vi "ProducerConsumerDAQ.vi"() -> ()   [LabVIEW 2014]
doc: "Use this template to build a user interface event handler design pattern. Use this pattern for dialog boxes and other user interfaces. You also can create and execute user-defined events that the VI can handle the same way as user interface events."
uses:
  subVIs/MasterState.ctl
  subVIs/SlaveStateData.ctl
  subVIs/SlaveState.ctl
  <vilib>/Utility/error.llb/DialogType.ctl
  <vilib>/DAQmx/create/channels.llb/DAQmx Create Channel (AI-Voltage-Basic).vi
  <vilib>/DAQmx/configure/timing.llb/DAQmx Timing (Sample Clock).vi
  <vilib>/DAQmx/read.llb/DAQmx Read (Analog Wfm 1Chan NSamp).vi
  <resource>/objmgr/daqmx.rc
panel:
  in  "File Path":path
  in  "Acquire Data":bool
  in  "Log Data":bool
  in  "File Comment":string
  in  "DAQ Parameters":T1={"physical channels"="", "maximum value"=5.0, "minimum value"=-5.0, "rate"=1000.0, "read period"=0.5} {"read period" format="%0.2f"; "rate" format="%0.2f"; "minimum value" format="%0.2f"; "maximum value" format="%0.2f"}
  out "Waveform Chart":waveform(dbl)(graph)
  in  "quit":bool
  # "V"
  # "V"
  # "Hz"
  # "s"
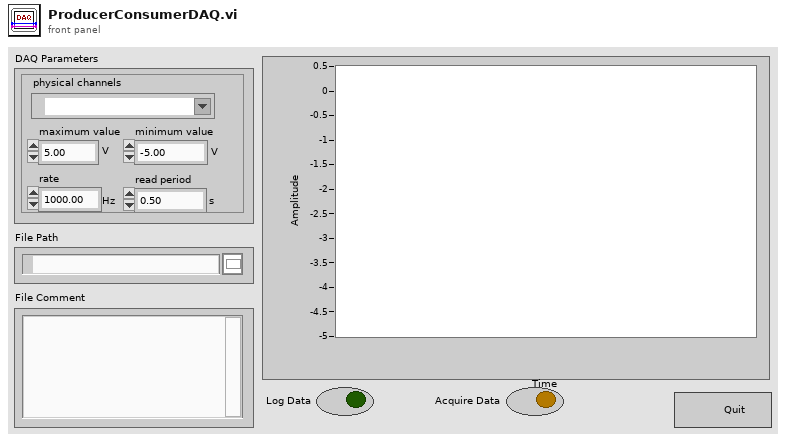
[diagram p1: front panel]
types:
  T1 = cluster{"physical channels":tag, "maximum value":dbl, "minimum value":dbl, "rate":dbl, "read period":dbl}
  T2 = typedef "SlaveState.ctl" = enum16{"Init", "Idle", "CheckError", "Finalize", "StartDAQ", "AcquireAndLog", "StopDAQ", "UpdateFile"}
  T3 = typedef "SlaveStateData.ctl" = cluster{"New State":T2, "DAQ Ref":refnum<k21>, "File Ref":refnum<file>}
  T4 = typedef "MasterState.ctl" = enum16{"Init", "Idle", "CheckError", "Finalize", "ConfigDAQ", "StartDAQ", "AcquireAndLog", "StopDAQ", "ClearDAQ", "OpenFile", "CloseFile"}
  T5 = typedef "DialogType.ctl" = u16
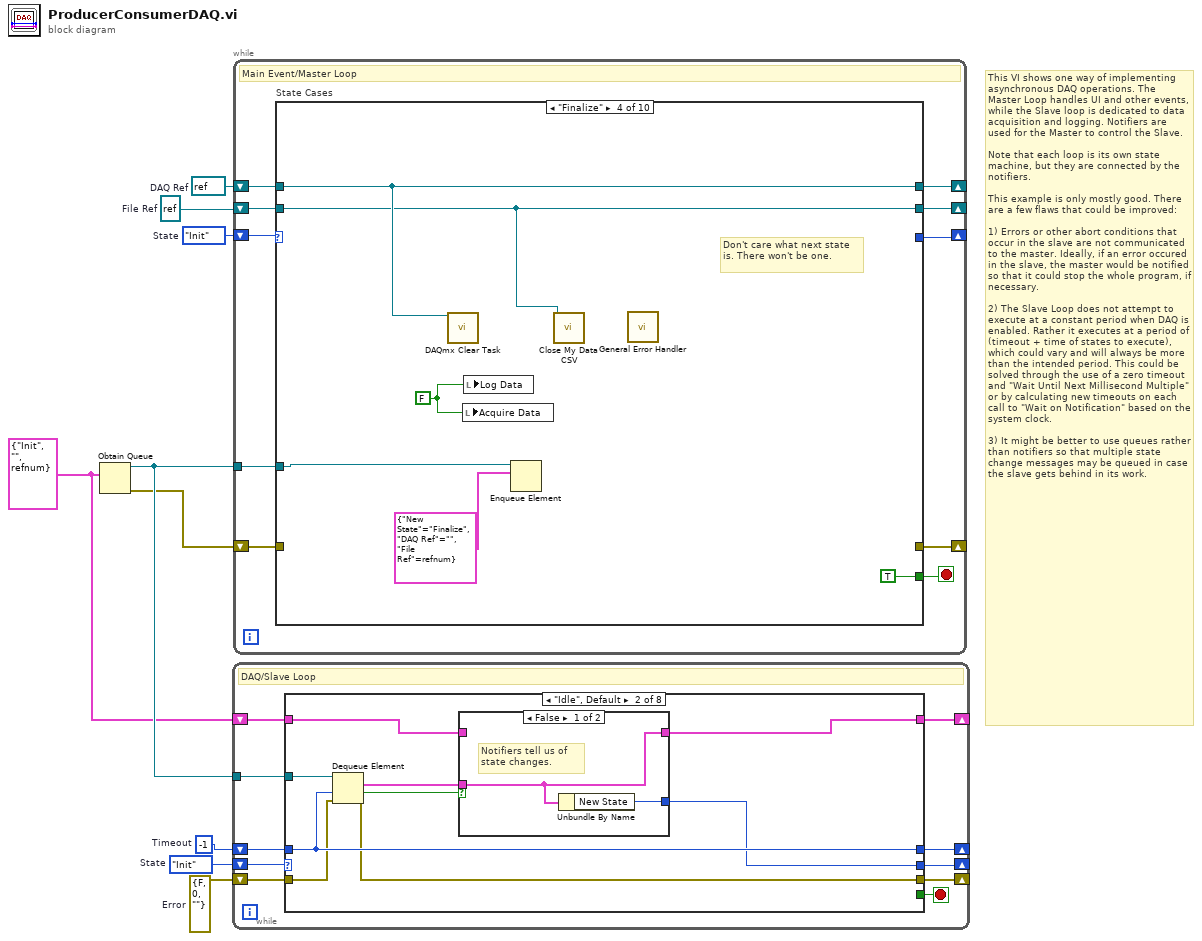
[diagram p0: block diagram]
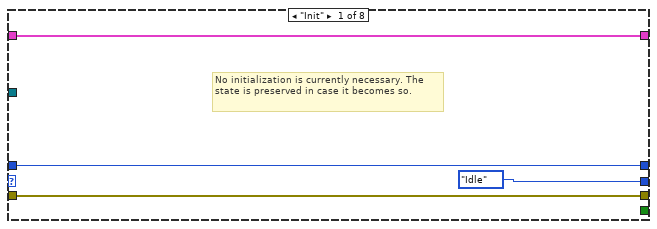
[diagram p2: hidden frame]
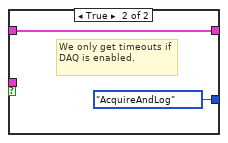
[diagram p3: hidden frame]
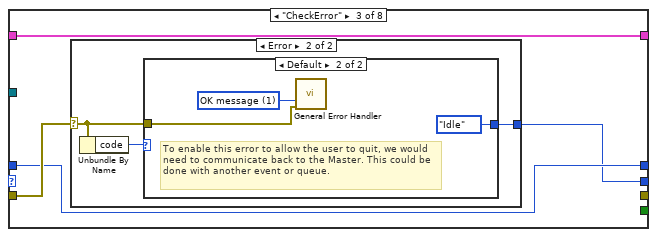
[diagram p4: hidden frame]
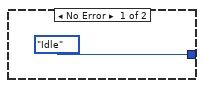
[diagram p5: hidden frame]
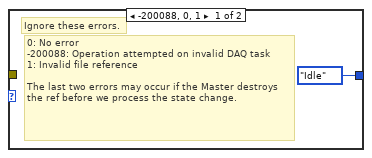
[diagram p6: hidden frame]
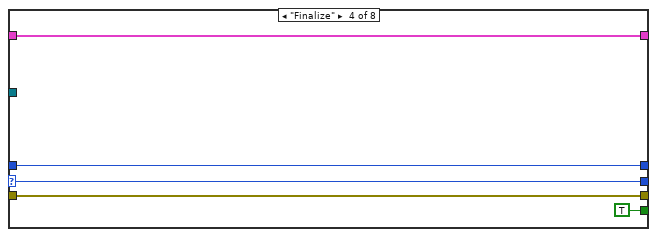
[diagram p7: hidden frame]
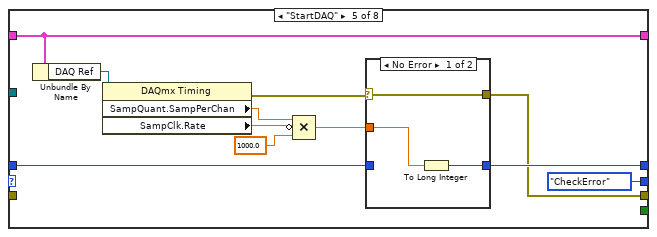
[diagram p8: hidden frame]
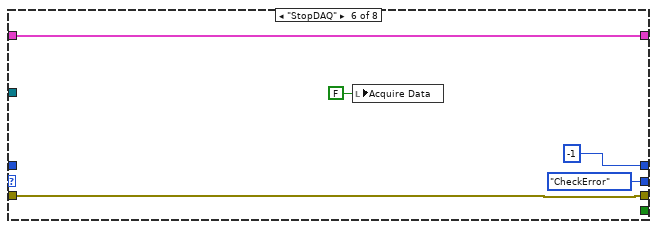
[diagram p10: hidden frame]
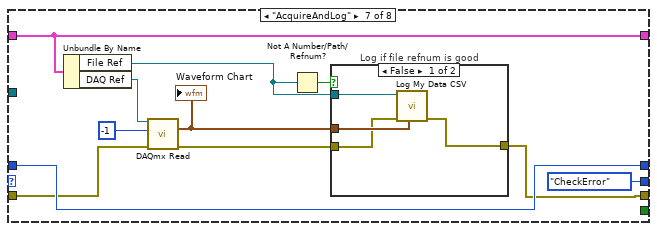
[diagram p11: hidden frame]
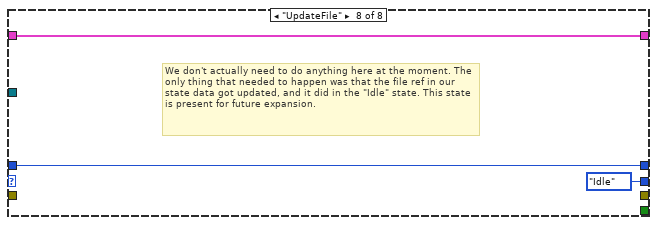
[diagram p13: hidden frame]
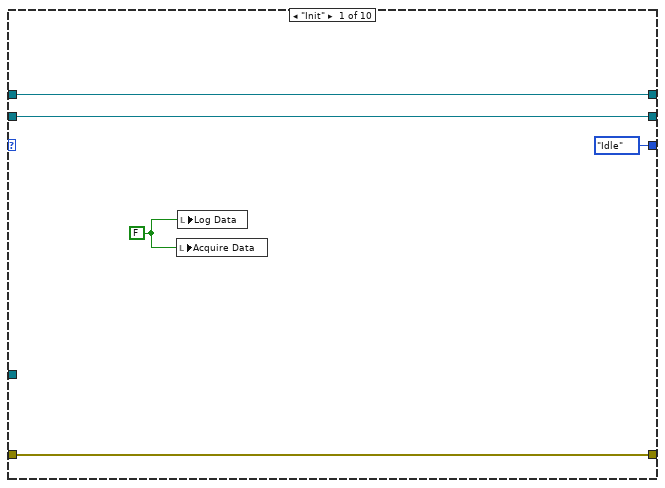
[diagram p14: hidden frame]
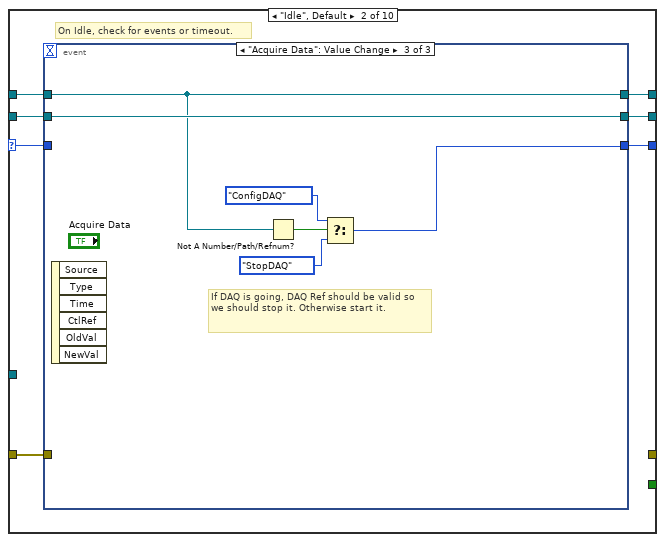
[diagram p15: hidden frame]
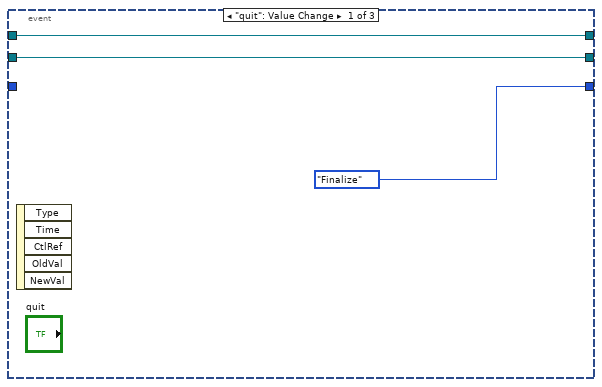
[diagram p16: hidden frame]
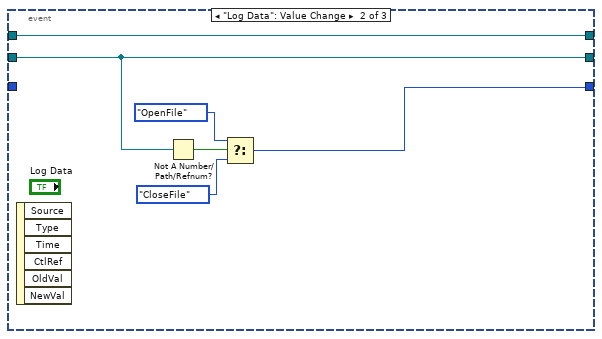
[diagram p17: hidden frame]
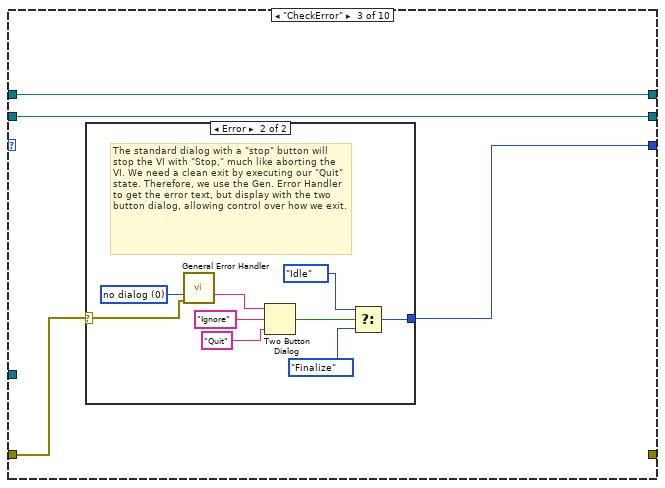
[diagram p18: hidden frame]
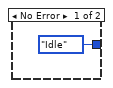
[diagram p19: hidden frame]
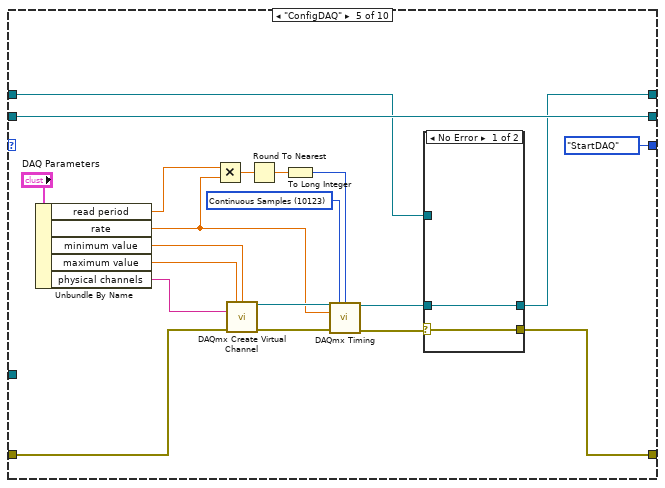
[diagram p20: hidden frame]
diagram:
  w1 = errorcluster {"status"=FALSE, "code"=0, "source"=""}  # Error
  w3 = -1  # Timeout
  w5 = SlaveState."Init"  # State
  w4 = T3 {"New State"=enum."Init", "DAQ Ref"="", "File Ref"=refnum}
  w7 = refnum<file> refnum  # File Ref
  w8 = refnum<k21> refnum  # DAQ Ref
  w9 = MasterState."Init"  # State
  # "This VI shows one way of implementing asynchronous DAQ operations. The Master Loop handles UI and other events, while the Slave loop is dedicated to data acquisition and logging. Notifiers are used for the Master to control the Slave.\n\nNote that each loop is its own state machine, but they are connected by the notifiers.\n\nThis example is only mostly good. There are a few flaws that could be improved:\n\n1) Errors or other abort conditions that occur in the slave are not communicated to the master. Ideally, if an error occured in the slave, the master would be notified so that it could stop the whole program, if necessary.\n\n2) The Slave Loop does not attempt to execute at a constant period when DAQ is enabled. Rather it executes at a period of (timeout + time of states to execute), which could vary and will always be more than the intended period. This could be solved through the use of a zero timeout and \"Wait Until Next Millisecond Multiple\" or by calculating new timeouts on each call to \"Wait on Notification\" based on the system clock.\n\n3) It might be better to use queues rather than notifiers so that multiple state change messages may be queued in case the slave gets behind in its work."
  n1 = Obtain Queue(element data type=w4) -> (queue out=w6:refnum<queue>, error out=w2:errorcluster)  [unwired: 4 in, 1 out]
  n2 = while {
    tunnel: w6 -> [w18]
    shift-right: [w17] -> _
    shift-left: w5 -> [w19]
    shift-right: [w13] -> _
    shift-left: w4 -> [w16]
    shift-right: [w14] -> _
    shift-left: w3 -> [w15]
    shift-right: [w11] -> _
    shift-left: w1 -> [w12]
    stop <- w10 stop-if-true
    # "DAQ/Slave Loop"
    n3 = case shown="\"Idle\", Default" w19 {
      selector: w19 -> [_ _ _ w50 _ _ _ _]
      tunnel: w18 -> [_ w32 _ _ _ _ _ _]
      tunnel: [SlaveState."Idle" ("New State") w25 w37 w50 SlaveState."CheckError" ("State") SlaveState."CheckError" ("State") SlaveState."CheckError" ("State") SlaveState."Idle" ("State")] -> w17
      tunnel: w16 -> [w21 w27 w40 w52 w61 w74 w79 w93]
      tunnel: w15 -> [w22 w31 w38 w51 w63 _ w80 w92]
      tunnel: [w22 w31 w38 w51 w64 -1 w80 w92] -> w14
      tunnel: [w21 w24 w40 w52 w61 w74 w79 w93] -> w13
      tunnel: w12 -> [w20 w29 w39 w49 _ w70 w77 _]
      tunnel: [w20 w30 _ w49 w62 w70 w76 _] -> w11
      tunnel: [_ _ _ TRUE _ _ _ _] -> w10
      frame "Init" {
        # "No initialization is currently necessary. The state is preserved in case it becomes so."
      }
      frame "Idle", Default {
        n4 = Dequeue Element(queue=w32, timeout in ms (-1)=w31, error in (no error)=w29) -> (element=w26:T3, timed out?=w28:bool, error out=w30:errorcluster)  [unwired: 1 out]
        n5 = case shown="False" w28 {
          tunnel: w27 -> [_ w36]
          tunnel: w26 -> [w33 _]
          tunnel: [w34 SlaveState."AcquireAndLog" ("New State")] -> w25
          tunnel: [w33 w36] -> w24
          frame False {
            # "Notifiers tell us of state changes."
            n6 = Unbundle By Name(w33) -> ("New State"=w34:T2)
          }
          frame True {
            # "We only get timeouts if DAQ is enabled."
          }
        }
      }
      frame "CheckError" {
        n7 = case shown="Error" w39 {
          selector: w39 -> [_ w43]
          tunnel: [SlaveState."Idle" ("State") w44] -> w37
          frame No Error {
          }
          frame Error {
            n8 = Unbundle By Name(w43) -> ("code"=w42:i32)
            n9 = case shown="Default" w42 {
              tunnel: [SlaveState."Idle" ("State") SlaveState."Idle" ("State")] -> w44
              tunnel: w43 -> [_ w47]
              frame -200088, 0, 1 {
                # "0: No error\n-200088: Operation attempted on invalid DAQ task\n1: Invalid file reference\n\nThe last two errors may occur if the Master destroys the ref before we process the state change."
                # "Ignore these errors."
              }
              frame Default {
                w48 = T5 1 items=["no dialog", "OK message", "continue or stop message", "OK message + warnings", "continue/stop + warnings"] ("type of dialog (OK msg:1)")
                # "To enable this error to allow the user to quit, we would need to communicate back to the Master. This could be done with another event or queue."
                n10 = call <vilib>:"General Error Handler.vi"("type of dialog (OK msg:1)"=w48, "error in (no error)"=w47) -> ()  [unwired: 9 in, 5 out]
              }
            }
          }
        }
      }
      frame "Finalize" {
      }
      frame "StartDAQ" {
        n11 = Unbundle By Name(w61) -> ("DAQ Ref"=w60:refnum<k21>)
        n12 = property class="DAQmx Timing"(reference=w60) -> (error out=w58:errorcluster, "SampQuant.SampPerChan"=w57:dbl, "SampClk.Rate"=w56:dbl)  [unwired: 1 in, 1 out]
        n13 = Compound Arithmetic op=MULTIPLY(w57, invert w56, 1000.0 ("value")) -> (w54:dbl)
        n14 = case shown="No Error" w58 {
          selector: w58 -> [w66 w69]
          tunnel: [w67 w68] -> w64
          tunnel: [w66 w69] -> w62
          tunnel: w63 -> [_ w68]
          tunnel: w54 -> [w65 _]
          frame No Error {
            n15 = To Long Integer(number=w65) -> (32bit integer=w67:i32)
          }
          frame Error {
          }
        }
      }
      frame "StopDAQ" {
        n16 = local write "Acquire Data"(FALSE ("Acquire Data")) -> ()
      }
      frame "AcquireAndLog" {
        n17 = Unbundle By Name(w79) -> ("File Ref"=w75:refnum<file>, "DAQ Ref"=w78:refnum<k21>)
        n18 = call-poly <vilib>:"DAQmx Read.vi"("task/channels in"=w78, "number of samples per channel"=-1, "error in"=w77) -> ("data"=w81:waveform(dbl), "error out"=w82:errorcluster)  [unwired: 10 in, 1 out]
        "Waveform Chart" <- w81
        n19 = Not A Number/Path/Refnum?(number/path/refnum=w75) -> (NaN/Path/Refnum?=w83:bool)
        n20 = case "Log if file refnum is good" shown="False" w83 {
          tunnel: w82 -> [w86 w90]
          tunnel: w75 -> [w89 _]
          tunnel: w81 -> [w88 _]
          tunnel: [w87 w90] -> w76
          frame False {
            n21 = call "Log My Data CSV.vi"("Data"=w88, "error in"=w86, "file refnum"=w89) -> ("error out"=w87:errorcluster)  [unwired: 7 in, 1 out]
          }
          frame True {
          }
        }
      }
      frame "UpdateFile" {
        # "We don't actually need to do anything here at the moment. The only thing that needed to happen was that the file ref in our state data got updated, and it did in the \"Idle\" state. This state is present for future expansion."
      }
    }
  }
  n22 = while {
    shift-right: [w102] -> _
    shift-left: w9 -> [w103]
    shift-right: [w101] -> _
    shift-left: w8 -> [w100]
    shift-right: [w99] -> _
    shift-left: w7 -> [w98]
    shift-right: [w97] -> _
    shift-left: w2 -> [w96]
    tunnel: w6 -> [w94]
    stop <- w95 stop-if-true
    # "Main Event/Master Loop"
    n23 = case "State Cases" shown="\"Finalize\"" w103 {
      selector: w103 -> [_ w115 _ _ _ _ _ _ _ _]
      tunnel: [MasterState."Idle" ("State") w114 w132 _ MasterState."StartDAQ" ("State") MasterState."CheckError" ("State") MasterState."ClearDAQ" ("State") MasterState."CheckError" ("State") MasterState."CheckError" ("State") MasterState."CheckError" ("State")] -> w102
      tunnel: [w108 w111 w134 w149 w161 w177 w191 refnum<k21> refnum ("DAQ Ref") w207 w233] -> w101
      tunnel: w100 -> [w108 w110 w134 w149 w162 w177 w191 w201 w207 w233]
      tunnel: [w107 w113 w133 w148 w170 w180 w198 w203 w218 w237] -> w99
      tunnel: w98 -> [w107 w112 w133 w148 w170 w180 w198 w203 w208 w240]
      tunnel: [w104 _ _ _ w159 w181 w193 w199 w217 w230] -> w97
      tunnel: w96 -> [w104 w109 w131 _ w151 w178 w190 w200 w214 w236]
      tunnel: [_ _ _ TRUE _ _ _ _ _ _] -> w95
      tunnel: w94 -> [_ _ _ w146 _ w185 w197 _ w211 w229]
      frame "Init" {
        w105 = FALSE
        n24 = local write "Acquire Data"(w105) -> ()
        n25 = local write "Log Data"(w105) -> ()
      }
      frame "Idle", Default {
        # "On Idle, check for events or timeout."
        # "States"
        n26 = event shown="[2] \"Acquire Data\": Value Change" {
          selector: _ -> [_ _ _]
          dyn-events: _ -> [_ _ _]
          timeout: _ -> [_ _ _]
          tunnel: w115 -> [_ _ _]
          tunnel: [MasterState."Finalize" ("State") w119 w125] -> w114
          tunnel: [w117 w122 w130] -> w113
          tunnel: w112 -> [w117 w122 w130]
          tunnel: [w118 w124 w128] -> w111
          tunnel: w110 -> [w118 w124 w128]
          tunnel: w109 -> [_ _ _]
          event "quit": Value Change {
            n27 = event-data() -> ()  [unwired: 1 in, 5 out]
          }
          event "Log Data": Value Change {
            n28 = event-data() -> ()  [unwired: 1 in, 6 out]
            n29 = Not A Number/Path/Refnum?(number/path/refnum=w122) -> (NaN/Path/Refnum?=w123:bool)
            n30 = Select(t=MasterState."OpenFile" ("State"), s=w123, f=MasterState."CloseFile" ("State")) -> (s? t:f=w119:T4)
          }
          event "Acquire Data": Value Change {
            # "If DAQ is going, DAQ Ref should be valid so we should stop it. Otherwise start it."
            n31 = event-data() -> ()  [unwired: 1 in, 6 out]
            n32 = Not A Number/Path/Refnum?(number/path/refnum=w128) -> (NaN/Path/Refnum?=w129:bool)
            n33 = Select(t=MasterState."ConfigDAQ" ("State"), s=w129, f=MasterState."StopDAQ" ("State")) -> (s? t:f=w125:T4)
          }
        }
      }
      frame "CheckError" {
        n34 = case shown="Error" w131 {
          selector: w131 -> [_ w136]
          tunnel: [MasterState."Idle" ("State") w137] -> w132
          frame No Error {
          }
          frame Error {
            w144 = T5 0 items=["no dialog", "OK message", "continue or stop message", "OK message + warnings", "continue/stop + warnings"] ("type of dialog (OK msg:1)")
            # "The standard dialog with a \"stop\" button will stop the VI with \"Stop,\" much like aborting the VI. We need a clean exit by executing our \"Quit\" state. Therefore, we use the Gen. Error Handler to get the error text, but display with the two button dialog, allowing control over how we exit."
            n35 = call <vilib>:"General Error Handler.vi"("type of dialog (OK msg:1)"=w144, "error in (no error)"=w136) -> ("message"=w143:string)  [unwired: 9 in, 4 out]
            n36 = Two Button Dialog(message=w143, 1:"Quit" ("F button name (\"Cancel\")"), 2:"Ignore" ("T button name (\"OK\")")) -> (T button?=w140:bool)
            n37 = Select(t=MasterState."Idle" ("State"), s=w140, f=MasterState."Finalize" ("State")) -> (s? t:f=w137:T4)
          }
        }
      }
      frame "Finalize" {
        w147 = FALSE
        # "Don't care what next state is. There won't be one."
        n38 = call <vilib>:"DAQmx Clear Task.vi"("task in"=w149) -> ()  [unwired: 14 in, 1 out]
        n39 = local write "Acquire Data"(w147) -> ()
        n40 = local write "Log Data"(w147) -> ()
        n41 = Enqueue Element(queue=w146, element=T3 {"New State"=enum."Finalize", "DAQ Ref"="", "File Ref"=refnum} ("notification")) -> ()  [unwired: 2 in, 3 out]
        n42 = call "Close My Data CSV.vi"("file refnum"=w148) -> ()  [unwired: 10 in, 1 out]
        n43 = call <vilib>:"General Error Handler.vi"() -> ()  [unwired: 11 in, 5 out]
      }
      frame "ConfigDAQ" {
        w167 = 10123 items=["Finite Samples"=10178, "Continuous Samples"=10123, "Hardware Timed Single Point"=12522] ("sample mode")
        n44 = Unbundle By Name("DAQ Parameters") -> ("read period"=w156:dbl, "rate"=w155:dbl, "minimum value"=w154:dbl, "maximum value"=w153:dbl, "physical channels"=w152:tag)
        n45 = Multiply(x=w156, y=w155) -> (x*y=w166:dbl)
        n46 = call-poly <vilib>:"DAQmx Create Virtual Channel.vi"("maximum value"=w153, "minimum value"=w154, "physical channels"=w152, "error in"=w151) -> ("task out"=w169:refnum<k21>, "error out"=w168:errorcluster)  [unwired: 10 in]
        n47 = Round To Nearest(number=w166) -> (nearest integer value=w165:dbl)
        n48 = To Long Integer(number=w165) -> (32bit integer=w164:i32)
        n49 = call-poly <vilib>:"DAQmx Timing.vi"("task/channels in"=w169, "sample mode"=w167, "samples per channel"=w164, "rate"=w155, "error in"=w168) -> ("task out"=w160:refnum<k21>, "error out"=w163:errorcluster)  [unwired: 9 in]
        n50 = case shown="No Error" w163 {
          selector: w163 -> [w171 w174]
          tunnel: w162 -> [_ w173]
          tunnel: [w172 w173] -> w161
          tunnel: w160 -> [w172 _]
          tunnel: [w171 w174] -> w159
          frame No Error {
          }
          frame Error {
          }
        }
      }
      frame "StartDAQ" {
        # "Set \"StartDAQ\" State on slave"
        n51 = call <vilib>:"DAQmx Start Task.vi"("task/channels in"=w177, "error in"=w178) -> ("error out"=w176:errorcluster)  [unwired: 12 in, 1 out]
        n52 = Bundle By Name(cluster=T3 {"New State"=enum."Init", "DAQ Ref"="", "File Ref"=refnum} ("notification"), "File Ref"=w180, "New State"=SlaveState."StartDAQ", "DAQ Ref"=w177) -> (w182:T3)
        n53 = Enqueue Element(queue=w185, element=w182, error in (no error)=w176) -> (error out=w181:errorcluster)  [unwired: 1 in, 2 out]
        n54 = case shown="No Error" w176 {
          tunnel: [TRUE FALSE] -> w175
          frame No Error {
          }
          frame Error {
          }
        }
        n55 = local write "Acquire Data"(w175) -> ()
      }
      frame "StopDAQ" {
        n56 = call <vilib>:"DAQmx Stop Task.vi"("task/channels in"=w191, "error in"=w190) -> ("error out"=w189:errorcluster)  [unwired: 12 in, 1 out]
        n57 = Bundle By Name(cluster=T3 {"New State"=enum."Init", "DAQ Ref"="", "File Ref"=refnum} ("notification"), "New State"=SlaveState."StopDAQ", "DAQ Ref"=refnum<k21> refnum) -> (w194:T3)
        n58 = Enqueue Element(queue=w197, element=w194, error in (no error)=w189) -> (error out=w193:errorcluster)  [unwired: 1 in, 2 out]
      }
      frame "ClearDAQ" {
        n59 = call <vilib>:"DAQmx Clear Task.vi"("task in"=w201, "error in"=w200) -> ("error out"=w199:errorcluster)  [unwired: 13 in]
      }
      frame "OpenFile" {
        # "Open new log file"
        # "Inform slave of new log file"
        n60 = Get Date/Time In Seconds() -> (seconds since 1Jan1904=w221:timestamp)
        n61 = call "Open My Data CSV.vi"("Comment"="File Comment", "Time Stamp"=w221, "error in"=w214, "file path"="File Path") -> ("error out"=w213:errorcluster, "refnum out"=w206:refnum<file>)  [unwired: 6 in]
        n62 = Bundle By Name(cluster=T3 {"New State"=enum."Init", "DAQ Ref"="", "File Ref"=refnum} ("notification"), "New State"=SlaveState."UpdateFile", "DAQ Ref"=w207, "File Ref"=w206) -> (w205:T3)
        n63 = Enqueue Element(queue=w211, element=w205, error in (no error)=w213) -> (error out=w212:errorcluster)  [unwired: 1 in, 2 out]
        n64 = case shown="No Error" w212 {
          selector: w212 -> [w223 w227]
          tunnel: [w224 w225] -> w218
          tunnel: w206 -> [w224 _]
          tunnel: [w223 w227] -> w217
          tunnel: [TRUE ("Log Data") FALSE ("Log Data")] -> w216
          tunnel: w208 -> [_ w225]
          frame No Error {
          }
          frame Error {
          }
        }
        n65 = local write "Log Data"(w216) -> ()
      }
      frame "CloseFile" {
        w232 = refnum<file> refnum  # File Ref
        w237 = refnum<file> refnum  # File Ref
        # "Close file"
        # "Inform slave of closed file"
        n66 = call "Close My Data CSV.vi"("error in"=w236, "file refnum"=w240) -> ("error out"=w231:errorcluster)  [unwired: 9 in]
        n67 = Bundle By Name(cluster=T3 {"New State"=enum."Init", "DAQ Ref"="", "File Ref"=refnum} ("notification"), "New State"=SlaveState."UpdateFile", "DAQ Ref"=w233, "File Ref"=w232) -> (w228:T3)
        n68 = Enqueue Element(queue=w229, element=w228, error in (no error)=w231) -> (error out=w230:errorcluster)  [unwired: 1 in, 2 out]
        n69 = local write "Log Data"(FALSE ("Log Data")) -> ()
      }
    }
  }
